vi "ENABLE.vi"(2 "error out 4":errorcluster, 3 "VISA resource name 4":refnum<visa-resource-name>) -> (0 "error out 5":errorcluster, 1 "VISA resource name 5":refnum<visa-resource-name>)   [LabVIEW 2017]
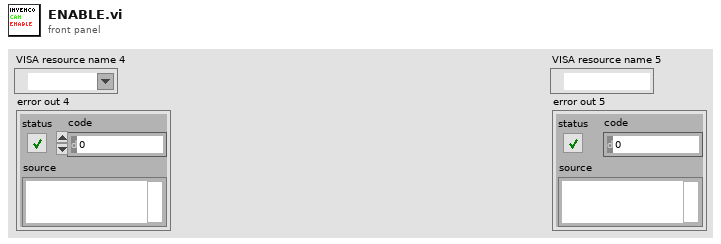
[diagram p1: front panel]
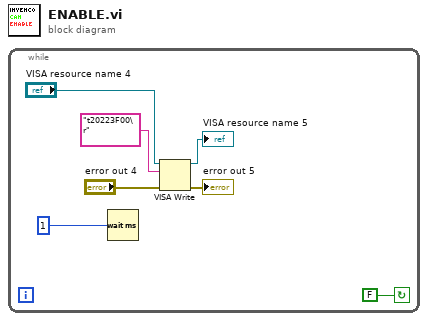
[diagram p0: block diagram]
diagram:
  n1 = while {
    stop <- FALSE continue-if-true
    n2 = Wait (ms)(milliseconds to wait=u32 1 ("millisecond multiple")) -> ()  [unwired: 1 out]
    n3 = VISA Write(VISA resource name="VISA resource name 4", write buffer="t20223F00\r", error in (no error)="error out 4") -> (VISA resource name out=→"VISA resource name 5":refnum<visa-resource-name>, error out=→"error out 5":errorcluster)  [unwired: 1 out]
  }
